vi "CohortShowElectd.vi"(8 "error in (no error)":errorcluster, 10 "Index":i32, 11 "Cohort in":refnum<class "Cohort.lvclass">) -> (0 "error out":errorcluster, 2 "Electrode":T1 {"Group #" format="%2d"; "Magnitude" format="%4.2f"}, 3 "Cohort out":refnum<class "Cohort.lvclass">)   [LabVIEW 2012, in "Cohort.lvclass"]
uses:
  Cohort.lvclass
  Cohort.lvclass/Cohort.ctl
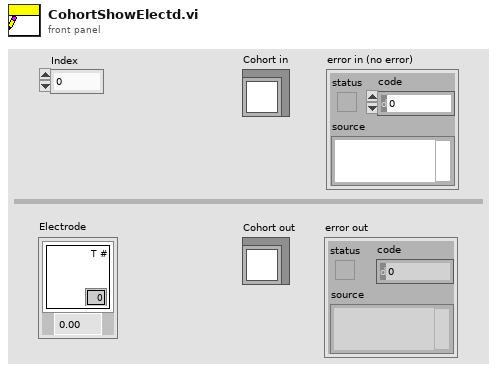
[diagram p1: front panel]
types:
  T1 = cluster{"T #":u8, "Magnitude":sgl, "Group #":dbl}
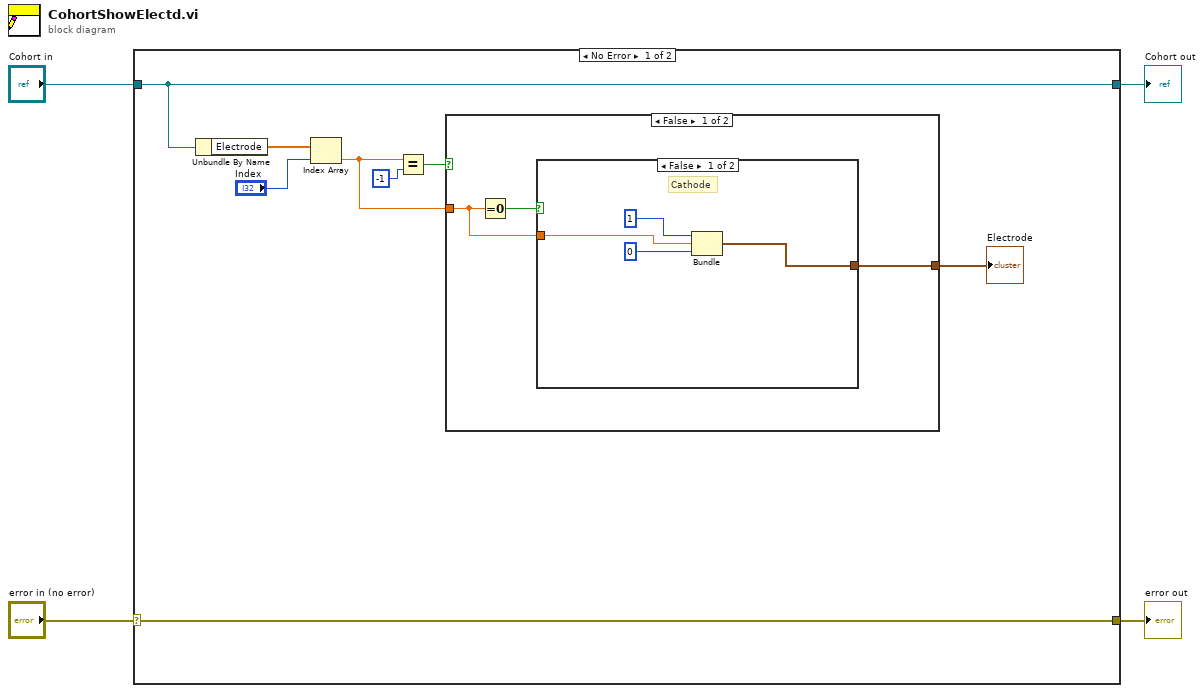
[diagram p0: block diagram]
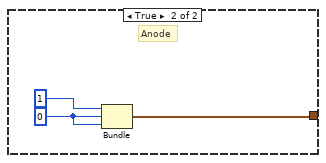
[diagram p2: hidden frame]
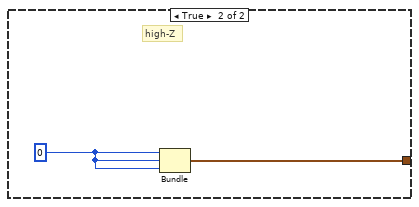
[diagram p3: hidden frame]
diagram:
  n1 = case shown="No Error" "error in (no error)" {
    selector: "error in (no error)" -> [w12 w25]
    tunnel: [w12 w25] -> w3
    tunnel: [w9 w26] -> w1
    tunnel: "Cohort in" -> [w9 w26]
    frame No Error {
      n2 = Unbundle By Name(w9) -> ("Electrode"=w11:sgl[])
      n3 = Index Array(array=w11, index="Index") -> (element=w5:sgl)
      n4 = Equal?(x=w5, y=-1) -> (x = y?=w7:bool)
      n5 = case shown="False" w7 {
        tunnel: [w14 w24] -> w6
        tunnel: w5 -> [w13 _]
        frame False {
          n6 = Equal To 0?(x=w13) -> (x = 0?=w15:bool)
          n7 = case shown="False" w15 {
            tunnel: [w16 w20] -> w14
            tunnel: w13 -> [w17 _]
            frame False {
              # "Cathode"
              n8 = Bundle(1, "Numeric"=w17, "T #"=u8 0) -> (w16:cluster{i32, "Numeric":sgl, "T #":u8})  [unwired: 1 in]
            }
            frame True {
              w22 = u8 0 ("T #")
              # "Anode"
              n9 = Bundle(1, "T #"=w22, "T #"=w22) -> (w20:cluster{i32, "T #":u8, "T #":u8})  [unwired: 1 in]
            }
          }
        }
        frame True {
          w23 = u8 0 ("T #")
          # "high-Z"
          n10 = Bundle("T #"=w23, "T #"=w23, "T #"=w23) -> (w24:cluster{"T #":u8, "T #":u8, "T #":u8})  [unwired: 1 in]
        }
      }
      "Electrode" <- w6
    }
    frame Error {
    }
  }
  "error out" <- w3
  "Cohort out" <- w1
